vi "niRFUtil WFM Scale Waveform (real wfm).vi"(4 "Scaling Waveform":T1 {"y" min=0 max=127 format="%.2f"; "dx" format="%^.2e"; "x0" format="%^.2e"}, 5 "Waveform In":T1 {"y" min=0 max=127 format="%.2f"; "dx" format="%^.2e"; "x0" format="%^.2e"}) -> (2 "Waveform Out":T1 {"y" min=0 max=127 format="%.2f"; "dx" format="%^.2e"; "x0" format="%^.2e"})   [LabVIEW 2015, in "niRFUtil.lvlib"]
doc: "(c) Copyright 2006, National Instruments, Inc. This VI may not be duplicated, sold, or distributed without written consent from National Instruments."
uses:
  niRFUtil.lvlib
  Includes/niRFUtil INC Real Waveform.ctl
  Includes/niRFUtil INC Real Array.ctl
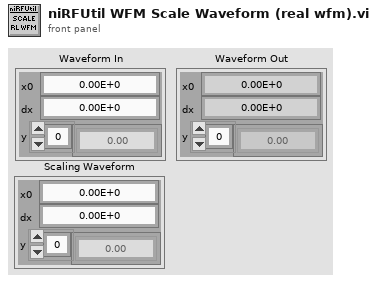
[diagram p1: front panel]
types:
  T1 = typedef "niRFUtil.lvlib/niRFUtil INC Real Waveform.ctl" = cluster{"x0":dbl, "dx":dbl, "y":T2}
  T2 = typedef "niRFUtil.lvlib/niRFUtil INC Real Array.ctl" = sgl[]
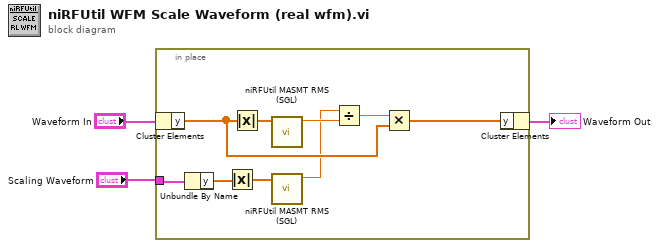
[diagram p0: block diagram]
diagram:
  n1 = in-place {
    in-place-border: "Scaling Waveform" -> [w7]
    n2 = in-place-cluster #1("Waveform In") -> ("y"=w11:T2)
    n3 = Unbundle By Name(w7) -> ("y"=w6:T2)
    n4 = Absolute Value(x=w6) -> (abs(x)=w5:T2)
    n5 = Absolute Value(x=w11) -> (abs(x)=w9:T2)
    n6 = call "niRFUtil MASMT RMS (SGL).vi"("X"=w9) -> ("rms"=w8:sgl)  [unwired: 9 in, 1 out]
    n7 = call "niRFUtil MASMT RMS (SGL).vi"("X"=w5) -> ("rms"=w4:sgl)  [unwired: 9 in, 1 out]
    n8 = Divide(x=w4, y=w8) -> (x/y=w12:sgl)
    n9 = Multiply(x=w12, y=w11) -> (x*y=w10:T2)
    n10 = in-place-cluster #1("y"=w10) -> (→"Waveform Out":T1)
  }
